vi "5 - Arduino.vi"() -> ()   [LabVIEW 2020]
uses:
  <vilib>/LabVIEW Interface for Arduino/Type Defs/Connection Type.ctl
  <vilib>/LabVIEW Interface for Arduino/Type Defs/Board Type.ctl
  <vilib>/LabVIEW Interface for Arduino/Type Defs/Pin Mode.ctl
  <vilib>/LabVIEW Interface for Arduino/LabVIEW Interface for Arduino.lvlib
panel:
  in  "Parar":bool
  in  "Saída 3":bool
  in  "VISA resource":refnum<visa-resource-name>
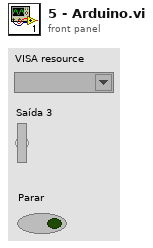
[diagram p1: front panel]
types:
  T1 = typedef "LabVIEW Interface for Arduino.lvlib/Board Type.ctl" = enum16{"Uno", "Dimuelanove w/Atmega 328", "Mega 2560"}
  T2 = typedef "LabVIEW Interface for Arduino.lvlib/Connection Type.ctl" = enum8{"USB / Serial", "XBEE", "BlueSmirf (Bluetooth)"}
  T3 = typedef "LabVIEW Interface for Arduino.lvlib/Arduino Resource.ctl" = cluster{"VISA resource":refnum<visa-resource-name>, "Board Type":T1, "Connection Type":enum8{"USB / Serial"}, "Bytes Per Packet (15)":u8}
  T4 = typedef "LabVIEW Interface for Arduino.lvlib/Pin Mode.ctl" = enum8{"Input", "Output"}
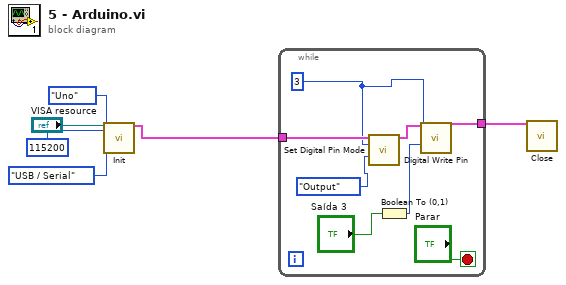
[diagram p0: block diagram]
diagram:
  n1 = call <vilib>:"Init.vi"("VISA resource"="VISA resource", "Baud Rate (115200)"=115200, "Board Type (Uno)"=Board_Type."Uno", "Connection Type (USB/Serial)"=Connection_Type."USB / Serial") -> ("Arduino Resource"=w1:T3)  [unwired: 14 in, 1 out]
  n2 = while {
    tunnel: [w11] -> w3
    tunnel: w1 -> [w10]
    stop <- "Parar" stop-if-true
    w7 = u8 3 ("Digital I/O Pin")
    n3 = call <vilib>:"Set Digital Pin Mode.vi"("Arduino Resource"=w10, "Digital I/O Pin"=w7, "Pin Mode (Input)"=Pin_Mode."Output") -> ("Arduino Resource"=w8:T3)  [unwired: 11 in, 1 out]
    n4 = Boolean To (0,1)(Boolean="Saída 3") -> (0, 1=w13:i16)
    n5 = call <vilib>:"Digital Write Pin.vi"("Arduino Resource"=w8, "Digital I/O Pin (0)"=w7, "Value (0)"=w13) -> ("Arduino Resource"=w11:T3)  [unwired: 11 in, 1 out]
  }
  n6 = call <vilib>:"Close.vi"("Arduino Resource"=w3) -> ()  [unwired: 14 in, 1 out]
